vi "DtAinContinuous.vi"() -> ()   [LabVIEW 2022 SP3]
doc: "The DtAinContinuous example demonstrates how to continuously acquire data from an analog input channel. This example runs continuously until either the Stop button is pressed or an error occurs."
uses:
  PolySubVIs/DtOLReadMultiple2D.vi
  PolySubVIs/DtOLTimingSetInput.vi
  PolySubVIs/DtCreateAinChan.vi
panel:
  in  "Start Button":bool
  in  "Device":string(combo)
  out "Acquired Data":dbl[][](graph)
  in  "Samples Per Channel":dbl=1000.0
  in  "Sample Rate":dbl=10000.0
  in  "Stop Button":bool
  in  "Channels":string="0"
  # "Continuous Analog Input Example"
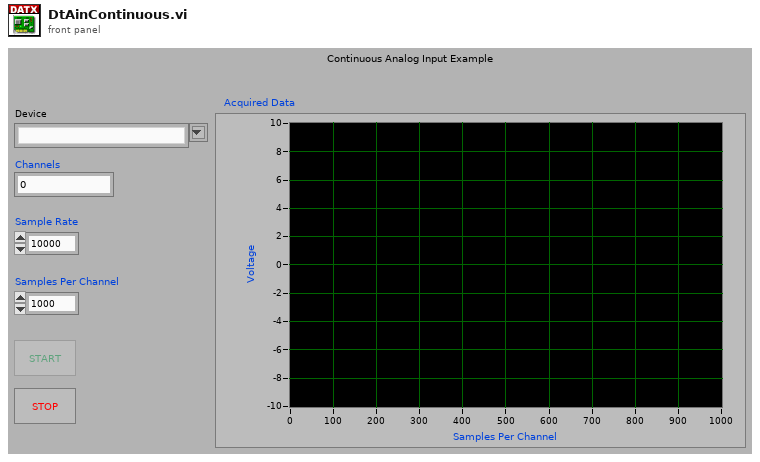
[diagram p1: front panel]
types:
  T1 = enum8{"Enabled", "Disabled", "Disabled and Grayed Out"}
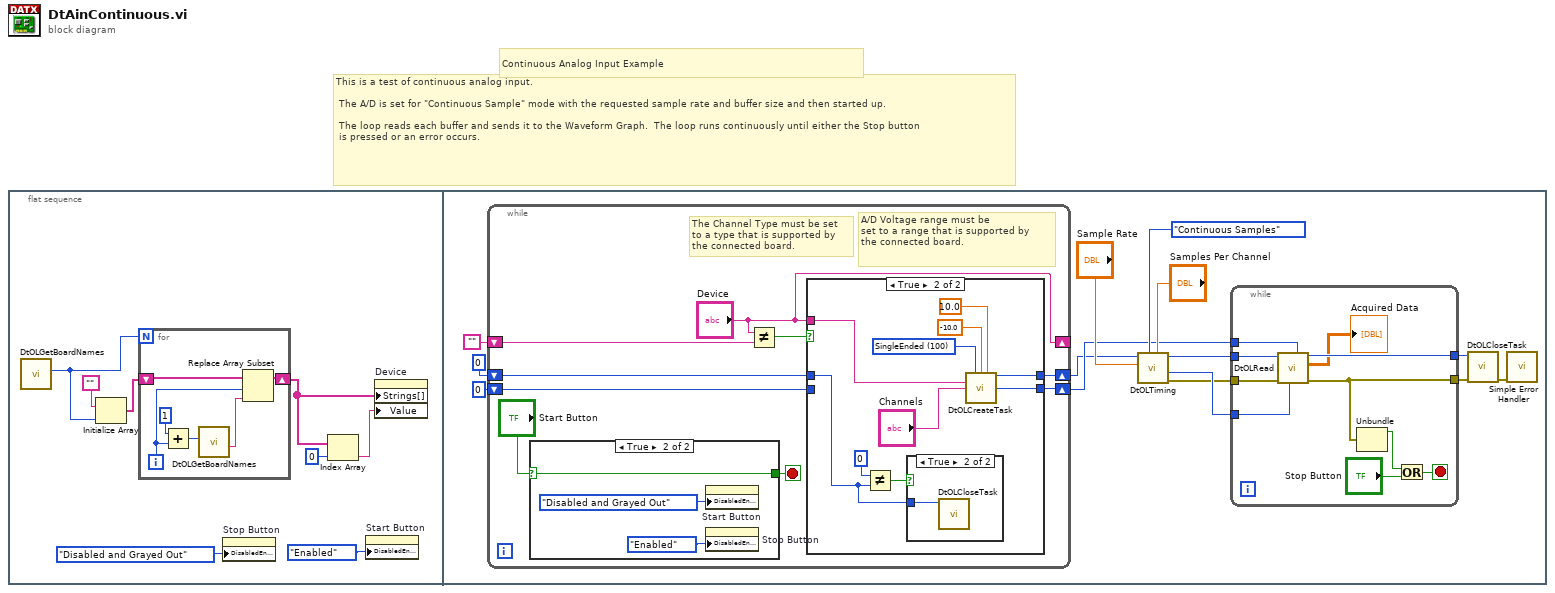
[diagram p0: block diagram]
diagram:
  # "Continuous Analog Input Example"
  # "This is a test of continuous analog input. \n\n The A/D is set for \"Continuous Sample\" mode with the requested sample rate and buffer size and then started up.\n\n The loop reads each buffer and sends it to the Waveform Graph.  The loop runs continuously until either the Stop button\n is pressed or an error occurs."
  n1 = flat-sequence {
    frame #0 {
      n2 = call "DtOLGetBoardNames.vi"() -> ("Number of boards"=w8:u32)  [unwired: 9 in, 2 out]
      n3 = Initialize Array("", w8) -> (w6:string[])
      n4 = for {
        N: w8 -> [_]
        shift-right: [w11] -> w3
        shift-left: w6 -> [w12]
        i -> [w10]
        n5 = Add(x=1, y=w10) -> (x+y=w14:i32)
        n6 = call "DtOLGetBoardNames.vi"("Select Board"=w14) -> ("Board Name"=w9:string)  [unwired: 8 in, 2 out]
        n7 = Replace Array Subset(array=w12, new element=w9, index=w10) -> (w11:string[])
      }
      n8 = property on="Stop Button" class="Bool"("DisabledEnum"=T1."Disabled and Grayed Out" ("Disabled")) -> ()  [unwired: 2 in, 2 out]
      n9 = Index Array(array=w3, index=0) -> (element=w4:string)
      n10 = property on="Start Button" class="Bool"("DisabledEnum"=T1."Enabled" ("Disabled")) -> ()  [unwired: 2 in, 2 out]
      n11 = property on="Device" class="CmbBox"("Strings[]"=w3, "Value"=w4) -> ()  [unwired: 2 in, 2 out]
    }
    frame #1 {
      n12 = while {
        shift-right: ["Device"] -> _
        shift-left: "" -> [w36]
        shift-right: [w33] -> w15
        shift-left: 0 ("Task out") -> [w34]
        shift-right: [w31] -> w16
        shift-left: u32 0 ("Actual Number of Channels") -> [w30]
        stop <- w32 stop-if-true
        # "The Channel Type must be set\nto a type that is supported by \nthe connected board."
        # "A/D Voltage range must be\nset to a range that is supported by \nthe connected board."
        n13 = case shown="True" "Start Button" {
          selector: "Start Button" -> [w38 w41]
          tunnel: [w38 w41] -> w32
          frame False {
          }
          frame True {
            n14 = property on="Start Button" class="Bool"("DisabledEnum"=T1."Disabled and Grayed Out" ("Disabled")) -> ()  [unwired: 2 in, 2 out]
            n15 = property on="Stop Button" class="Bool"("DisabledEnum"=T1."Enabled" ("Disabled")) -> ()  [unwired: 2 in, 2 out]
          }
        }
        n16 = Not Equal?(x="Device", y=w36) -> (x != y?=w37:bool)
        n17 = case shown="True" w37 {
          tunnel: "Device" -> [_ w50]
          tunnel: [w43 w49] -> w33
          tunnel: w34 -> [w43 w46]
          tunnel: [w42 w44] -> w31
          tunnel: w30 -> [w42 _]
          frame False {
          }
          frame True {
            w51 = 100 items=["SingleEnded"=100, "Differential"=101] ("Channel Type")
            n18 = Not Equal?(x=0, y=w46) -> (x != y?=w47:bool)
            n19 = case shown="True" w47 {
              tunnel: w46 -> [_ w54]
              frame False {
              }
              frame True {
                n20 = call "DtOLCloseTask.vi"("Task in"=w54) -> ()  [unwired: 10 in, 1 out]
              }
            }
            n21 = call-poly "DtOLCreateTask.vi"("Channel Type"=w51, "Range Min"=-10.0, "Range Max"=10.0, "Board Name"=w50, "Channel"="Channels") -> ("Task out"=w49:i32, "Actual Number of Channels"=w44:u32)  [unwired: 8 in, 1 out]
          }
        }
      }
      n22 = call-poly "DtOLTiming.vi"("Samples Per Channel"="Samples Per Channel", "Sample Mode"=enum16{"Finite Samples", "Continuous Samples"}."Continuous Samples", "Sample Freq (Hz)"="Sample Rate", "Task in"=w15) -> ("error out"=w27:errorcluster, "Buffer Size"=w28:u32, "Task out"=w26:i32)  [unwired: 4 in, 1 out]
      n23 = while {
        tunnel: w27 -> [w64]
        tunnel: [w63] -> w24
        tunnel: [w62] -> w25
        tunnel: w26 -> [w59]
        tunnel: w16 -> [w56]
        tunnel: w28 -> [w55]
        stop <- w58 stop-if-true
        n24 = call-poly "DtOLRead.vi"("Number Chan to Read"=w56, "Buffer size"=w55, "error in (no error)"=w64, "Task in"=w59) -> ("error out"=w62:errorcluster, "2D Data out"=→"Acquired Data":dbl[][], "Task out"=w63:i32)  [unwired: 3 in, 2 out]
        n25 = Unbundle(w62) -> ("status"=w61:bool)  [unwired: 2 out]
        n26 = Or(x=w61, y="Stop Button") -> (x .or. y?=w58:bool)
      }
      n27 = call "DtOLCloseTask.vi"("Error in"=w25, "Task in"=w24) -> ("Error Out"=w22:errorcluster)  [unwired: 9 in]
      n28 = call <vilib>:"Simple Error Handler.vi"("error in (no error)"=w22) -> ()  [unwired: 4 in, 5 out]
    }
  }
